vi "fdafsdfsf.vi"() -> ()   [LabVIEW 2014]
uses:
  <vilib>/Utility/config.llb/Read Key (String).vi
  <vilib>/Utility/config.llb/NI_LVConfig.lvlib
panel:
  out "string":string
  in  "stop":bool
  in  "MUX S.n.":string
  in  "BTbatt":bool
  in  "BTch0":bool
  in  "BTch4":bool
  in  "BTch3":bool
  in  "BTch2":bool
  in  "BTch1":bool
  out "ext.cmd":string=" -b"
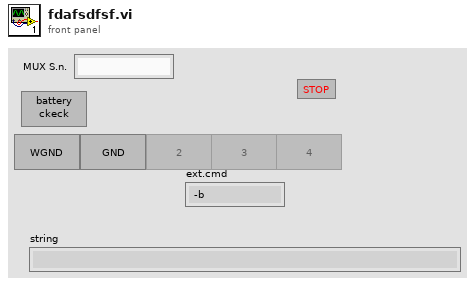
[diagram p1: front panel]
types:
  T1 = typedef "NI_LVConfig.lvlib/Config Data RefNum.ctl" = refnum<k1>
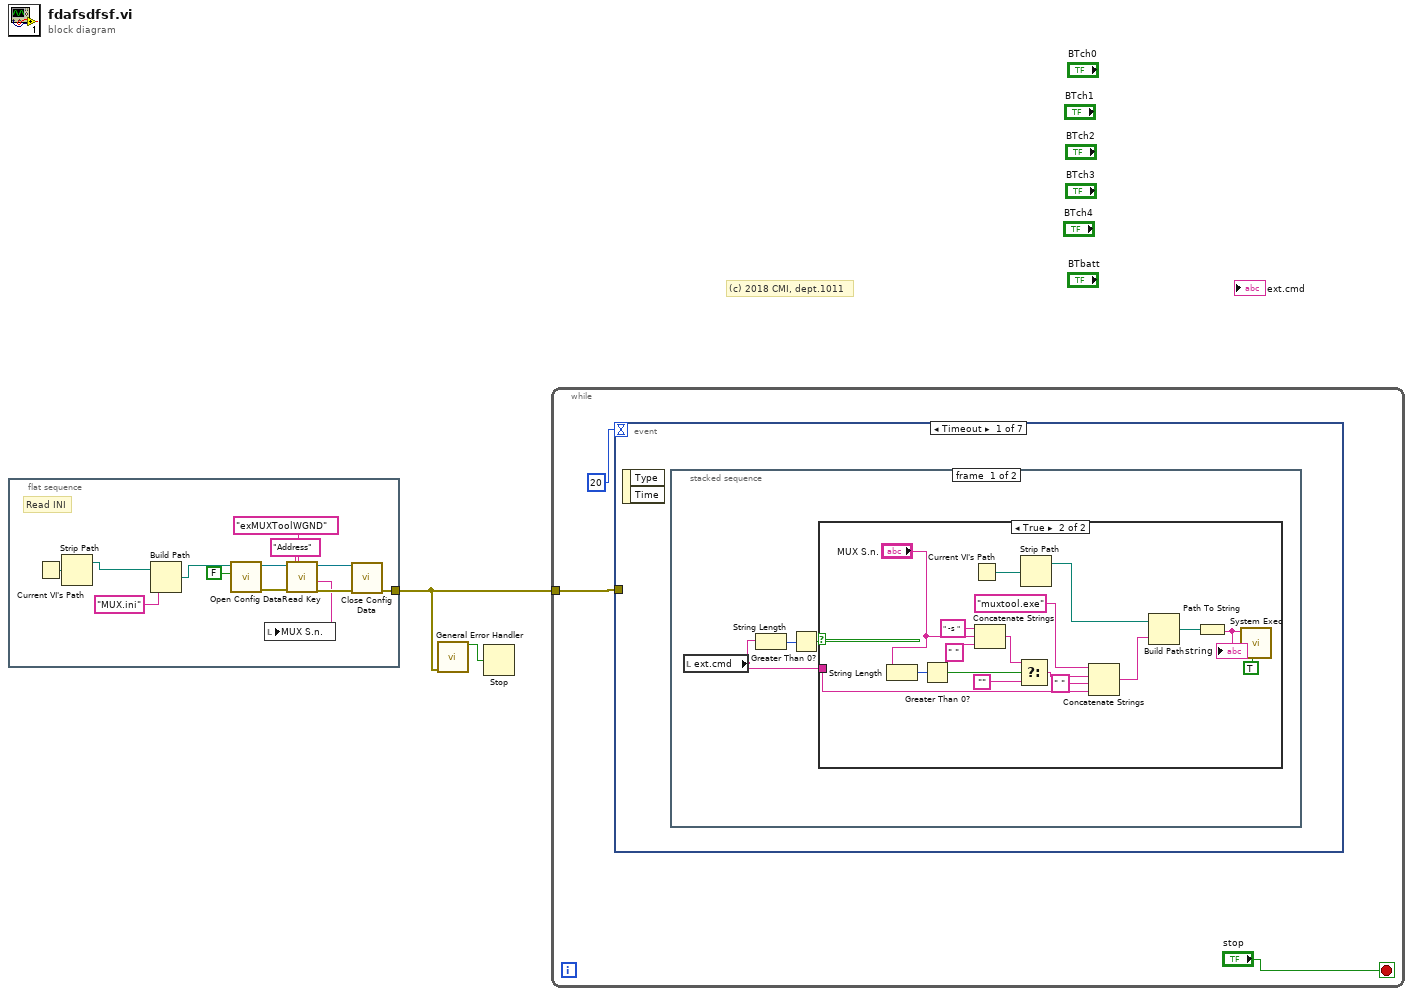
[diagram p0: block diagram]
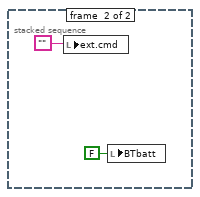
[diagram p3: hidden frame]
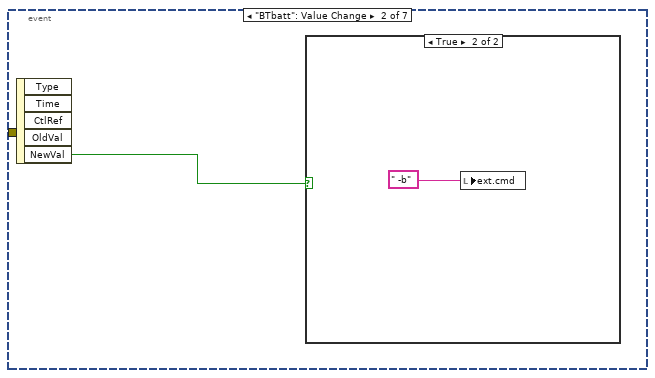
[diagram p4: hidden frame]
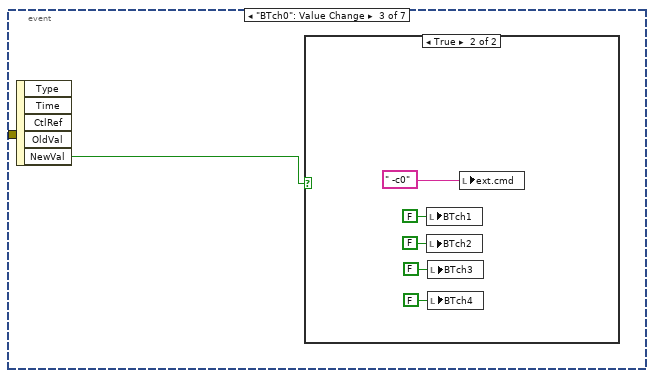
[diagram p6: hidden frame]
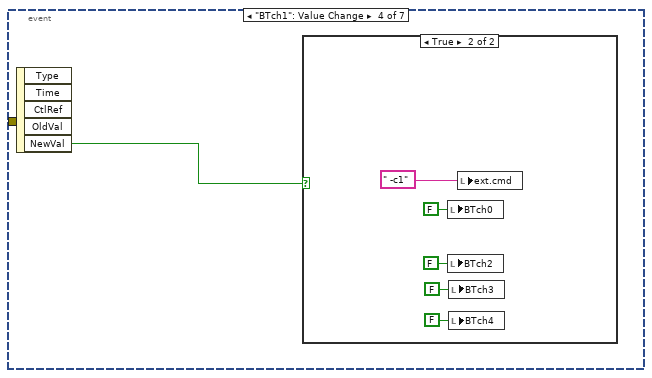
[diagram p8: hidden frame]
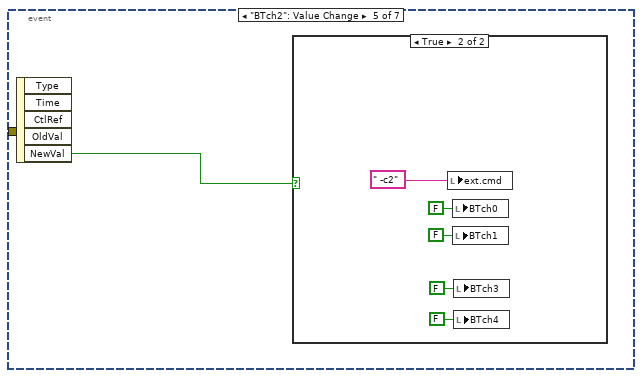
[diagram p10: hidden frame]
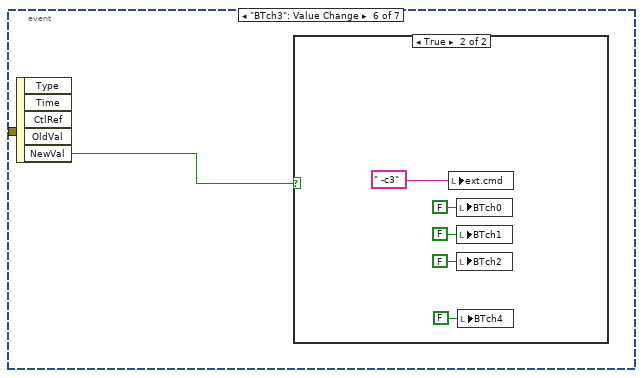
[diagram p12: hidden frame]
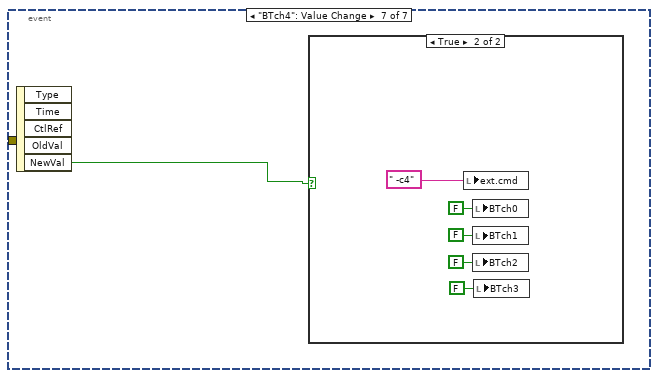
[diagram p14: hidden frame]
diagram:
  # "(c) 2018 CMI, dept.1011"
  n1 = flat-sequence {
    tunnel: [w6] -> w1
    frame #0 {
      # "Read INI"
      n2 = Current VI's Path() -> (path=w4:path)
      n3 = Strip Path(path=w4) -> (stripped path=w3:path)  [unwired: 1 out]
      n4 = Build Path(base path=w3, name or relative path="MUX.ini") -> (appended path=w14:path)
      n5 = call <vilib>:"Open Config Data.vi"("create file if necessary (T)"=FALSE, "configuration file path"=w14) -> ("error out"=w12:errorcluster, "refnum"=w5:T1)  [unwired: 7 in, 1 out]
      n6 = call-poly <vilib>:"Read Key.vi"("section"="exMUXToolWGND", "error in (no error)"=w12, "key"="Address", "refnum"=w5) -> ("error out"=w8:errorcluster, "value"=w7:string, "refnum out"=w9:T1)  [unwired: 4 in, 1 out]
      n7 = local write "MUX S.n."(w7) -> ()
      n8 = call <vilib>:"Close Config Data.vi"("error in (no error)"=w8, "refnum"=w9) -> ("error out"=w6:errorcluster)  [unwired: 8 in, 1 out]
    }
  }
  n9 = call <vilib>:"General Error Handler.vi"("error in (no error)"=w1) -> ("error?"=w2:bool)  [unwired: 10 in, 4 out]
  n10 = Stop(stop? (T)=w2) -> ()
  n11 = while {
    tunnel: w1 -> [w17]
    stop <- "stop" stop-if-true
    n12 = event shown="[0] Timeout" {
      selector: _ -> [_ _ _ _ _ _ _]
      dyn-events: _ -> [_ _ _ _ _ _ _]
      timeout: 20 -> [_ _ _ _ _ _ _]
      tunnel: w17 -> [_ _ _ _ _ _ _]
      event Timeout {
        n13 = event-data() -> ()  [unwired: 1 in, 2 out]
        n14 = stacked-sequence {
          frame #0 {
            n15 = local read "ext.cmd"() -> (w19:string)
            n16 = String Length(string=w19) -> (length=w20:i32)
            n17 = Greater Than 0?(x=w20) -> (x > 0?=w21:bool)
            n18 = case shown="True" w21 {
              tunnel: w19 -> [_ w31]
              frame False {
              }
              frame True {
                n19 = String Length(string="MUX S.n.") -> (length=w28:i32)
                n20 = Greater Than 0?(x=w28) -> (x > 0?=w27:bool)
                n21 = Current VI's Path() -> (path=w36:path)
                n22 = Concatenate Strings(" -s " ("string"), "MUX S.n.", " " ("string")) -> (w24:string)
                n23 = Select(t=w24, s=w27, f="") -> (s? t:f=w29:string)
                n24 = Strip Path(path=w36) -> (stripped path=w35:path)  [unwired: 1 out]
                n25 = Concatenate Strings("muxtool.exe" ("name or relative path"), w29, " " ("string"), w31) -> (w32:string)
                n26 = Build Path(base path=w35, name or relative path=w32) -> (appended path=w38:path)
                n27 = Path To String(path=w38) -> (string=w37:string)
                "string" <- w37
                n28 = call <vilib>:"System Exec.vi"("run minimized? (F)"=TRUE, "command line"=w37) -> ()  [unwired: 6 in, 4 out]
              }
            }
          }
          frame #1 {
            n29 = local write "ext.cmd"("") -> ()
            n30 = local write "BTbatt"(FALSE ("BTch0")) -> ()
          }
        }
      }
      event "BTbatt": Value Change {
        n31 = event-data() -> ("NewVal"=w41:bool)  [unwired: 1 in, 4 out]
        n32 = case shown="True" w41 {
          frame False {
          }
          frame True {
            n33 = local write "ext.cmd"(" -b" ("string")) -> ()
          }
        }
      }
      event "BTch0": Value Change {
        n34 = event-data() -> ("NewVal"=w43:bool)  [unwired: 1 in, 4 out]
        n35 = case shown="True" w43 {
          frame False {
          }
          frame True {
            n36 = local write "BTch1"(FALSE ("BTch0")) -> ()
            n37 = local write "BTch2"(FALSE ("BTch0")) -> ()
            n38 = local write "BTch3"(FALSE ("BTch0")) -> ()
            n39 = local write "BTch4"(FALSE ("BTch0")) -> ()
            n40 = local write "ext.cmd"(" -c0" ("string")) -> ()
          }
        }
      }
      event "BTch1": Value Change {
        n41 = event-data() -> ("NewVal"=w49:bool)  [unwired: 1 in, 4 out]
        n42 = case shown="True" w49 {
          frame False {
          }
          frame True {
            n43 = local write "BTch0"(FALSE ("BTch0")) -> ()
            n44 = local write "BTch2"(FALSE ("BTch0")) -> ()
            n45 = local write "BTch3"(FALSE ("BTch0")) -> ()
            n46 = local write "BTch4"(FALSE ("BTch0")) -> ()
            n47 = local write "ext.cmd"(" -c1" ("string")) -> ()
          }
        }
      }
      event "BTch2": Value Change {
        n48 = event-data() -> ("NewVal"=w55:bool)  [unwired: 1 in, 4 out]
        n49 = case shown="True" w55 {
          frame False {
          }
          frame True {
            n50 = local write "ext.cmd"(" -c2" ("string")) -> ()
            n51 = local write "BTch0"(FALSE ("BTch0")) -> ()
            n52 = local write "BTch1"(FALSE ("BTch0")) -> ()
            n53 = local write "BTch3"(FALSE ("BTch0")) -> ()
            n54 = local write "BTch4"(FALSE ("BTch0")) -> ()
          }
        }
      }
      event "BTch3": Value Change {
        n55 = event-data() -> ("NewVal"=w61:bool)  [unwired: 1 in, 4 out]
        n56 = case shown="True" w61 {
          frame False {
          }
          frame True {
            n57 = local write "ext.cmd"(" -c3" ("string")) -> ()
            n58 = local write "BTch0"(FALSE ("BTch0")) -> ()
            n59 = local write "BTch1"(FALSE ("BTch0")) -> ()
            n60 = local write "BTch2"(FALSE ("BTch0")) -> ()
            n61 = local write "BTch4"(FALSE ("BTch0")) -> ()
          }
        }
      }
      event "BTch4": Value Change {
        n62 = event-data() -> ("NewVal"=w67:bool)  [unwired: 1 in, 4 out]
        n63 = case shown="True" w67 {
          frame False {
          }
          frame True {
            n64 = local write "ext.cmd"(" -c4" ("string")) -> ()
            n65 = local write "BTch0"(FALSE ("BTch0")) -> ()
            n66 = local write "BTch1"(FALSE ("BTch0")) -> ()
            n67 = local write "BTch2"(FALSE ("BTch0")) -> ()
            n68 = local write "BTch3"(FALSE ("BTch0")) -> ()
          }
        }
      }
    }
  }
